vi "create db readback string.vi"(8 "error in (no error)":errorcluster, 11 "beamline readbacks":T1) -> (0 "error out 2":errorcluster, 3 "arry of readback strings":string)   [LabVIEW 2016]
doc: "Takes readback data and creates a string containing all of the data"
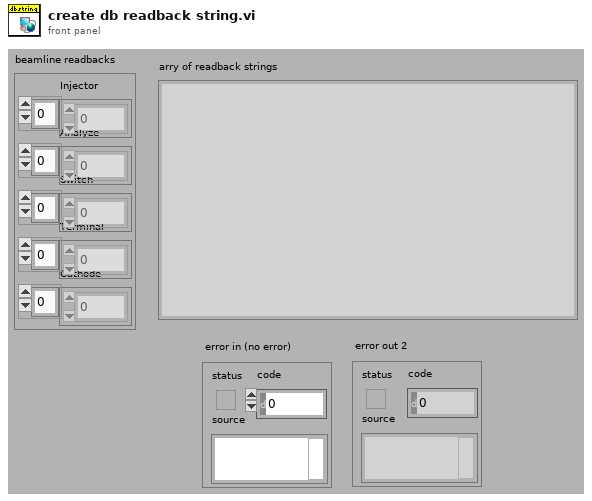
[diagram p1: front panel]
types:
  T1 = cluster{"Injector":dbl[], "Analyze":dbl[], "Switch":dbl[], "Terminal":dbl[], "Cathode":dbl[]}
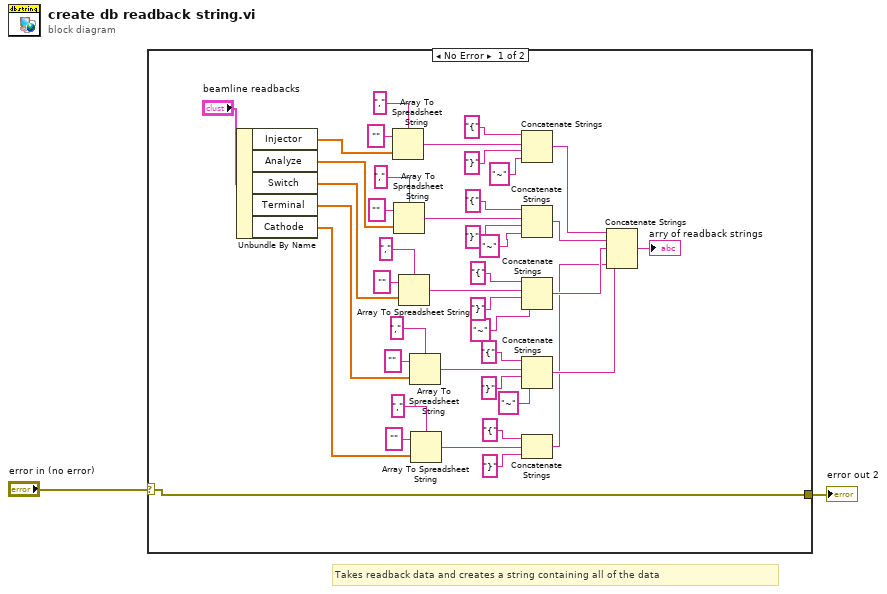
[diagram p0: block diagram]
diagram:
  # "Takes readback data and creates a string containing all of the data"
  n1 = case shown="No Error" "error in (no error)" {
    selector: "error in (no error)" -> [w3 w45]
    tunnel: [w3 w45] -> w1
    frame No Error {
      n2 = Unbundle By Name("beamline readbacks") -> ("Injector"=w44:dbl[], "Analyze"=w18:dbl[], "Switch"=w17:dbl[], "Terminal"=w16:dbl[], "Cathode"=w15:dbl[])
      n3 = Array To Spreadsheet String(delimiter (Tab)=",", array=w44, 3:"" ("format string")) -> (spreadsheet string=w39:string)
      n4 = Array To Spreadsheet String(delimiter (Tab)=",", array=w18, 3:"" ("format string")) -> (spreadsheet string=w38:string)
      n5 = Array To Spreadsheet String(delimiter (Tab)=",", array=w17, 3:"" ("format string")) -> (spreadsheet string=w29:string)
      n6 = Array To Spreadsheet String(delimiter (Tab)=",", array=w16, 3:"" ("format string")) -> (spreadsheet string=w28:string)
      n7 = Array To Spreadsheet String(delimiter (Tab)=",", array=w15, 3:"" ("format string")) -> (spreadsheet string=w19:string)
      n8 = Concatenate Strings("{" ("string"), w39, "}" ("string"), "~" ("string")) -> (w9:string)
      n9 = Concatenate Strings("{" ("string"), w38, "}" ("string"), "~" ("string")) -> (w8:string)
      n10 = Concatenate Strings("{" ("string"), w29, "}" ("string"), "~" ("string")) -> (w7:string)
      n11 = Concatenate Strings("{" ("string"), w28, "}" ("string"), "~" ("string")) -> (w6:string)
      n12 = Concatenate Strings("{" ("string"), w19, "}" ("string")) -> (w5:string)
      n13 = Concatenate Strings(w9, w8, w7, w6, w5) -> (→"arry of readback strings":string)
    }
    frame Error {
    }
  }
  "error out 2" <- w1
